vi "Rohde & Schwarz VNA Read Sweep Time.vi"(6 "Channel":i8=1 min=1 max=99 step=1, 7 "Rohde & Schwarz VNA":T1, 8 "error in (no error)":errorcluster, 11 "VISA Resource Name":refnum<visa-resource-name>) -> (0 "error out":errorcluster, 2 "Sweep Time, s":dbl=3000.0, 3 "dup VISA Resource Name":refnum<visa-resource-name>)   [LabVIEW 2011]
doc: "This Vi for the HP8753B Network Analyzer is used to set averaging, smoothing, and the IF bandwidth."
uses:
  TypeDefs/Rohde & Schwarz VNA Instrument Info.ctl
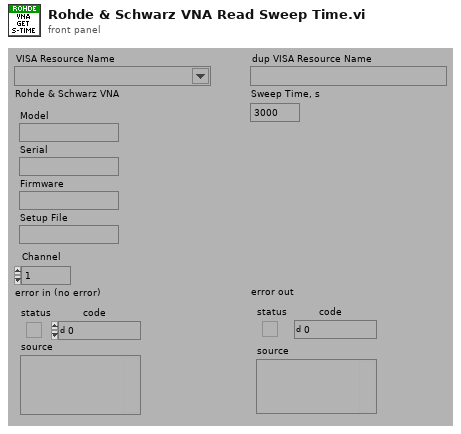
[diagram p1: front panel]
types:
  T1 = typedef "Rohde & Schwarz VNA Instrument Info.ctl" = cluster{"Model":string, "Serial":string, "Firmware":string, "Setup File":string}
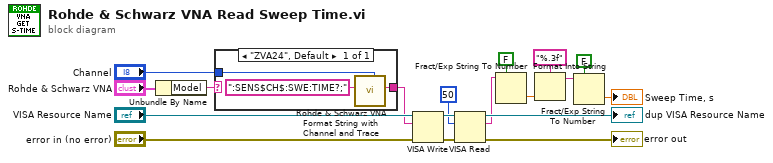
[diagram p0: block diagram]
diagram:
  n1 = Unbundle By Name("Rohde & Schwarz VNA") -> ("Model"=w1:string)
  n2 = case shown="\"ZVA24\", Default" w1 {
    tunnel: [w20] -> w4
    tunnel: "Channel" -> [w19]
    frame "ZVA24", Default {
      n3 = call "Rohde & Schwarz VNA Format String with Channel and Trace.vi"("Trace"=w19, "String"=":SENS$CH$:SWE:TIME?;") -> ("String Out"=w20:string)  [unwired: 1 in, 6 out]
    }
  }
  n4 = VISA Write(VISA resource name="VISA Resource Name", write buffer=w4, error in (no error)="error in (no error)") -> (VISA resource name out=w16:refnum<visa-resource-name>, error out=w12:errorcluster)  [unwired: 1 out]
  n5 = VISA Read(VISA resource name=w16, byte count=u32 50, error in (no error)=w12) -> (VISA resource name out=→"dup VISA Resource Name":refnum<visa-resource-name>, read buffer=w7:string, error out=→"error out":errorcluster)  [unwired: 1 out]
  n6 = Fract/Exp String To Number(use system decimal point (T)=FALSE, string=w7) -> (number=w10:dbl)  [unwired: 3 out]
  n7 = Format Into String(format string="%.3f", w10) -> (resulting string=w9:string)  [unwired: 2 in, 1 out]
  n8 = Fract/Exp String To Number(use system decimal point (T)=FALSE, string=w9) -> (number=→"Sweep Time, s":dbl)  [unwired: 3 out]
